vi "MB relay Configuration.vi"() -> ()   [LabVIEW 2016]
uses:
  APIs/type defs/baudrate.ctl
  <vilib>/Instr/_visa.llb/VISA Configure Serial Port (Instr).vi
  <vilib>/ErrorRing/Error Ring.xnode
  APIs/public/RELAYS Write the Baudrate.vi
  APIs/MB _relays.lvlib
panel:
  out "RelayBoard Infor":T1
  in  "stop":bool
  out "Response Log(HEX)":string
  in  "Refactory":bool
  in  "Scan Dev":bool
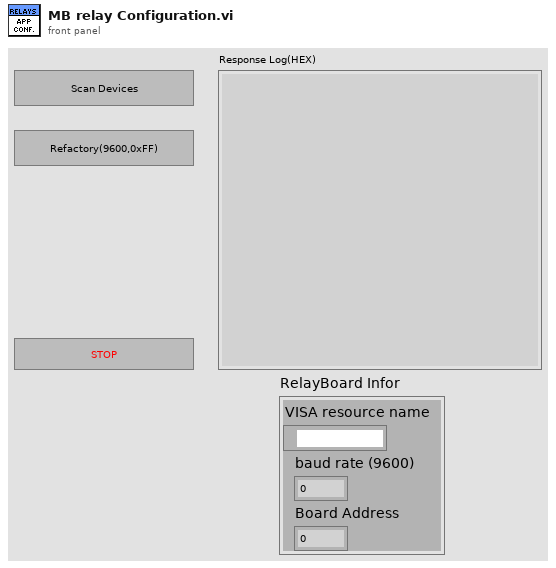
[diagram p1: front panel]
types:
  T1 = cluster{"VISA resource name":refnum<visa-resource-name>, "baud rate (9600)":u32, "Board Address":u8}
  T2 = typedef "MB _relays.lvlib/baudrate.ctl" = u8
  T3 = cluster{"VISA resource name":refnum<visa-resource-name>, "Board Address":u8, "baudrate(9600)":T2}
  T4 = typedef "Relay Board Infor.ctl" = cluster{"VISA resource name":refnum<visa-resource-name>, "Board Address":u8, "baudrate(9600)":T2}
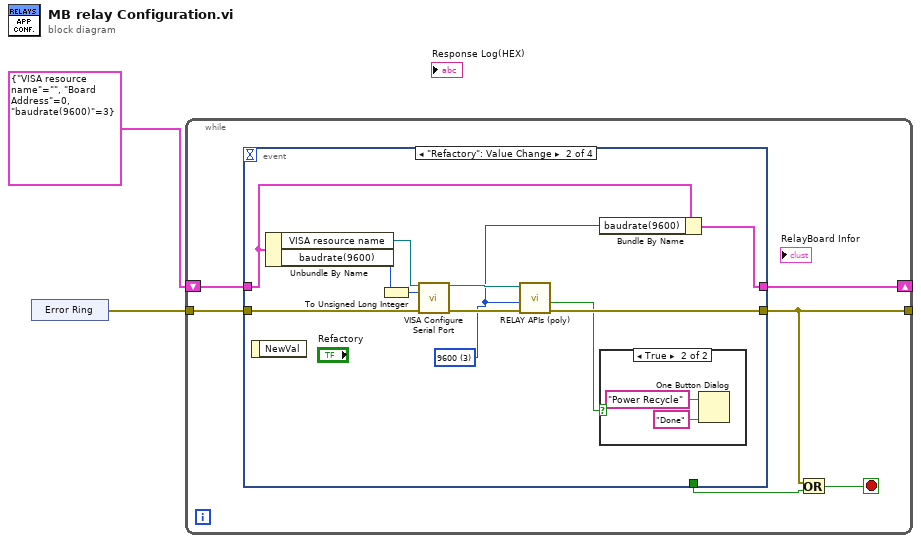
[diagram p0: block diagram]
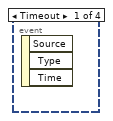
[diagram p2: hidden frame]
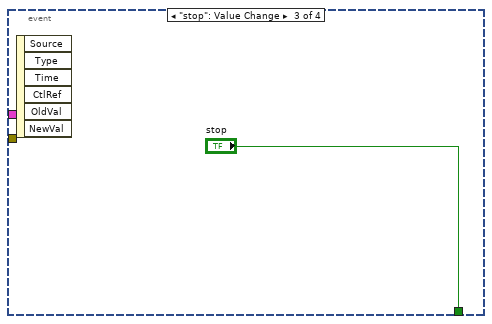
[diagram p4: hidden frame]
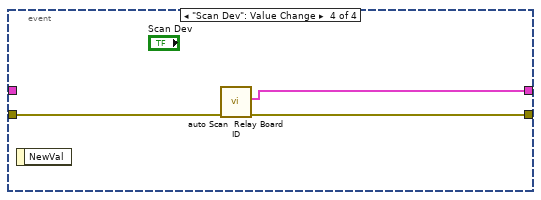
[diagram p5: hidden frame]
diagram:
  n1 = xnode "Error Ring"() -> ("error out"=w1:errorcluster)
  n2 = while {
    shift-right: [w8] -> _
    shift-left: T3 {"VISA resource name"="", "Board Address"=0, "baudrate(9600)"=3} ("RelayBoard Infor") -> [w7]
    tunnel: w1 -> [w6]
    tunnel: [w3] -> _
    stop <- w5 stop-if-true
    n3 = event shown="[1] \"Refactory\": Value Change" {
      selector: _ -> [_ _ _ _]
      dyn-events: _ -> [_ _ _ _]
      timeout: _ -> [_ _ _ _]
      tunnel: [_ _ "stop" _] -> w4
      tunnel: [_ w19 _ w23] -> w8
      tunnel: w7 -> [_ w14 _ _]
      tunnel: w6 -> [_ w18 _ w25]
      tunnel: [_ w10 _ w24] -> w3
      event Timeout {
        n4 = event-data() -> ()  [unwired: 1 in, 3 out]
      }
      event "Refactory": Value Change {
        w15 = T2 3 items=["4800"=2, "9600"=3, "19200"=4] ("baudrate")
        n5 = event-data() -> ()  [unwired: 1 in, 1 out]
        n6 = Unbundle By Name(w14) -> ("VISA resource name"=w13:refnum<visa-resource-name>, "baudrate(9600)"=w11:T2)
        n7 = To Unsigned Long Integer(number=w11) -> (unsigned 32bit integer=w12:u32)
        n8 = call-poly "VISA Configure Serial Port"("VISA resource name"=w13, "baud rate (9600)"=w12, "error in (no error)"=w18) -> ("VISA resource name out"=w17:refnum<visa-resource-name>, "error out"=w16:errorcluster)  [unwired: 11 in]
        n9 = call-poly "RELAY APIs (poly).vi"("error in (no error)"=w16, "baudrate"=w15, "VISA resource name"=w17) -> ("error out"=w10:errorcluster, "success?"=w9:bool)  [unwired: 5 in, 2 out]
        n10 = Bundle By Name(cluster=w14, "baudrate(9600)"=w15) -> (w19:T4)
        n11 = case shown="True" w9 {
          frame False {
          }
          frame True {
            n12 = One Button Dialog(message="Power Recycle", button name ("OK")="Done") -> ()  [unwired: 1 out]
          }
        }
      }
      event "stop": Value Change {
        n13 = event-data() -> ()  [unwired: 1 in, 6 out]
      }
      event "Scan Dev": Value Change {
        n14 = event-data() -> ()  [unwired: 1 in, 1 out]
        n15 = call "auto Scan  Relay Board ID.vi"("error in (no error)"=w25) -> ("error out"=w24:errorcluster, "RelayBoard Infor"=w23:T4)  [unwired: 9 in]
      }
    }
    n16 = Or(x=w3, y=w4) -> (x .or. y?=w5:bool)
  }
